vi "Emballage_BDD_choix_Config_Where.vi"(4 "Nom_Colonne":string="No_Valve_FAS", 6 "NewVal":u16, 7 "OldVal":u16, 8 "entrée d'erreur (pas d'erreur)":errorcluster, 9 "CtlRef":refnum<vi>, 10 "referenceWhere valeur":refnum<vi>, 11 "Array colonne":refnum<vi>) -> (0 "sortie d'erreur":errorcluster)   [LabVIEW 2020]
uses:
  Modules/FS/60_FS_Controles/60_FS_SetGet.ctl
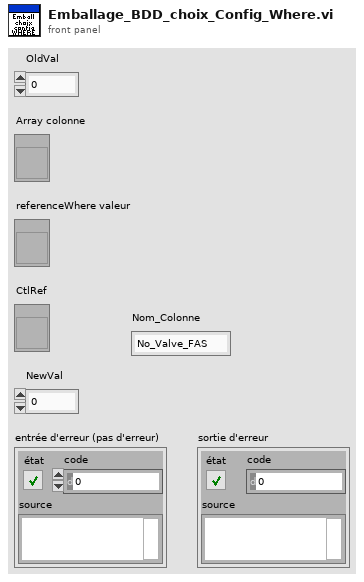
[diagram p1: front panel]
types:
  T1 = typedef "60_FS_SetGet.ctl" = enum16{"set", "get"}
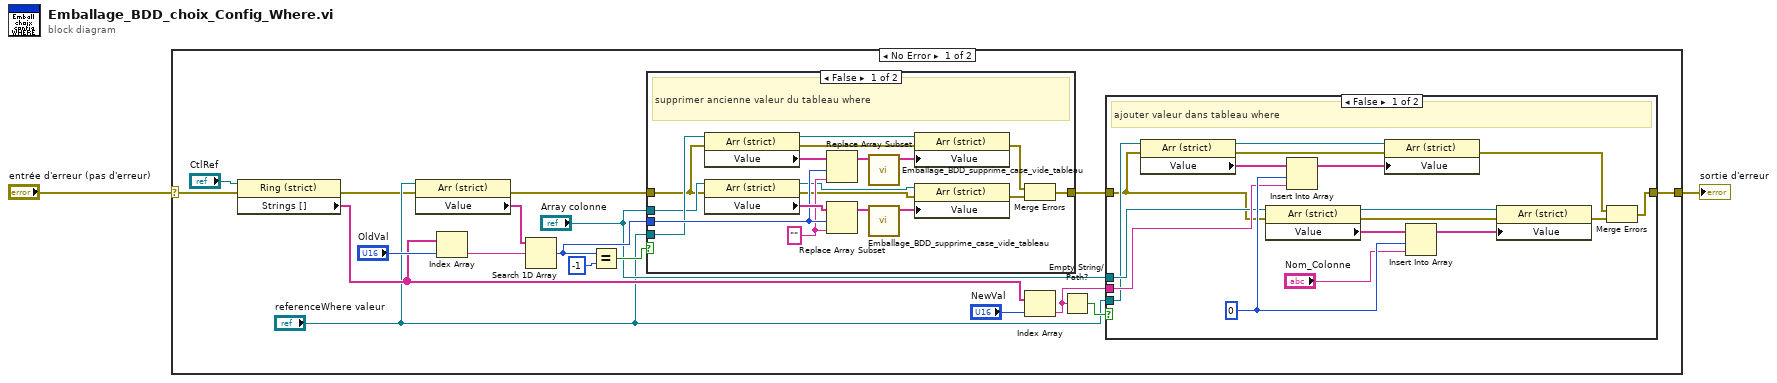
[diagram p0: block diagram]
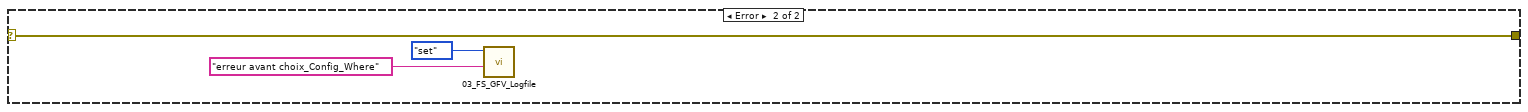
[diagram p4: hidden frame]
diagram:
  n1 = case shown="No Error" "entrée d'erreur (pas d'erreur)" {
    selector: "entrée d'erreur (pas d'erreur)" -> [w4 w60]
    tunnel: [w3 w60] -> w1
    frame No Error {
      n2 = property class="Ring (strict)"(reference="CtlRef", error in=w4) -> (error out=w6:errorcluster, "Strings []"=w11:string[])  [unwired: 1 out]
      n3 = property class="Arr (strict)"(reference="referenceWhere valeur", error in=w6) -> (error out=w5:errorcluster, "Value"=w18:string[])  [unwired: 1 out]
      n4 = Index Array(array=w11, index="OldVal") -> (element=w15:string)
      n5 = Search 1D Array(1D array=w18, element=w15) -> (index of element=w19:i32)  [unwired: 1 in]
      n6 = Equal?(x=w19, y=-1) -> (x = y?=w17:bool)
      n7 = case shown="False" w17 {
        tunnel: w19 -> [w36 _]
        tunnel: w5 -> [w24 w39]
        tunnel: [w23 w39] -> w20
        tunnel: "referenceWhere valeur" -> [w30 _]
        tunnel: "Array colonne" -> [w29 _]
        frame False {
          w35 = "" ("nouvel élément/sous-tableau")
          # "supprimer ancienne valeur du tableau where"
          n8 = property class="Arr (strict)"(reference=w30, error in=w24) -> (reference out=w28:refnum<vi>, error out=w27:errorcluster, "Value"=w38:string[])
          n9 = property class="Arr (strict)"(reference=w29, error in=w24) -> (reference out=w26:refnum<vi>, error out=w25:errorcluster, "Value"=w37:string[])
          n10 = Replace Array Subset(array=w38, new element=w35, index=w36) -> (w32:string[])
          n11 = Replace Array Subset(array=w37, new element=w35, index=w36) -> (w34:string[])
          n12 = call "Emballage_BDD_supprime_case_vide_tableau.vi"("Tableau IN"=w32) -> ("Tableau OUT"=w31:string[])  [unwired: 10 in]
          n13 = call "Emballage_BDD_supprime_case_vide_tableau.vi"("Tableau IN"=w34) -> ("Tableau OUT"=w33:string[])  [unwired: 10 in]
          n14 = property class="Arr (strict)"(reference=w28, error in=w27, "Value"=w31) -> (error out=w22:errorcluster)  [unwired: 1 out]
          n15 = property class="Arr (strict)"(reference=w26, error in=w25, "Value"=w33) -> (error out=w21:errorcluster)  [unwired: 1 out]
          n16 = Merge Errors(w22, w21) -> (w23:errorcluster)
        }
        frame True {
          # "si pas trouver => rien faire"
        }
      }
      n17 = Index Array(array=w11, index="NewVal") -> (element=w14:string)
      n18 = Empty String/Path?(string/path=w14) -> (empty?=w13:bool)
      n19 = case shown="False" w13 {
        tunnel: w14 -> [w50 _]
        tunnel: w20 -> [w43 w57]
        tunnel: [w42 w57] -> w3
        tunnel: "Array colonne" -> [w49 _]
        tunnel: "referenceWhere valeur" -> [w48 _]
        frame False {
          w52 = 0 ("indice")
          # "ajouter valeur dans tableau where"
          n20 = property class="Arr (strict)"(reference=w48, error in=w43) -> (reference out=w47:refnum<vi>, error out=w44:errorcluster, "Value"=w54:string[])
          n21 = property class="Arr (strict)"(reference=w49, error in=w43) -> (reference out=w46:refnum<vi>, error out=w45:errorcluster, "Value"=w55:string[])
          n22 = Insert Into Array(array=w54, index=w52, new element=w50) -> (w53:string[])
          n23 = property class="Arr (strict)"(reference=w47, error in=w44, "Value"=w53) -> (error out=w41:errorcluster)  [unwired: 1 out]
          n24 = Insert Into Array(array=w55, index=w52, new element="Nom_Colonne") -> (w56:string[])
          n25 = property class="Arr (strict)"(reference=w46, error in=w45, "Value"=w56) -> (error out=w40:errorcluster)  [unwired: 1 out]
          n26 = Merge Errors(w41, w40) -> (w42:errorcluster)
        }
        frame True {
          # "si élément actuelle est nul => rien faire"
        }
      }
    }
    frame Error {
      n27 = call "03_FS_GFV_Logfile.vi"("Chaîne"="erreur avant choix_Config_Where", "States"=60_FS_SetGet."set") -> ()  [unwired: 8 in, 2 out]
    }
  }
  "sortie d'erreur" <- w1
